vi "Apply Default.vi"(11 "Timestamp in":refnum<class "Timestamp.lvclass">) -> (3 "Timestamp out":refnum<class "Timestamp.lvclass">)   [LabVIEW 2020, in "Conditum.lvlib" / "Columns.lvlib" / "Timestamp.lvclass"]
uses:
  Timestamp.lvclass
  Timestamp.lvclass/Timestamp.ctl
  Type/Type.lvclass
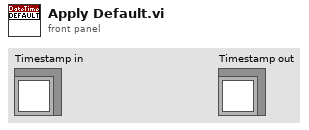
[diagram p1: front panel]
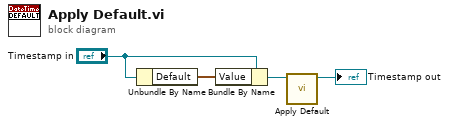
[diagram p0: block diagram]
diagram:
  n1 = Unbundle By Name("Timestamp in") -> ("Default"=w4:timestamp)
  n2 = Bundle By Name(cluster="Timestamp in", "Value"=w4) -> (w3:refnum<class "Timestamp.lvclass">)
  n3 = call-parent "Apply Default.vi"("Type in"=w3) -> ("Type out"=→"Timestamp out":refnum<class "Timestamp.lvclass">)  [unwired: 10 in]
